vi "Stop Core.vi"(10 "final error code":i32, 11 "Error Reporter in":refnum<class "Error Reporter.lvclass">) -> (3 "Error Reporter out":refnum<class "Error Reporter.lvclass">)   [LabVIEW 2024, in "Error Reporting Actor.lvlib" / "Error Reporter.lvlib" / "Error Reporter.lvclass"]
doc: "<p>(<strong>Filename</strong>: <span class=\"dnl\">Actor Framework.lvlib:Actor.lvclass:Stop Core.vi</span>)</p>\n<p>Defines what the actor does before it stops. Use the <strong>final error code</strong> input to determine whether the actor shut down in response to an error.</p>\n<p>By default, this method passes the Stop message along to all <a href=\"nihelplauncher://docs/csh?context=lvcore_lvcomm_af_launch_nested_actor\">auto-stop nested actors</a>. A descendant class may override this method to define additional behavior, such as shutting down any processes the actor initiated in its override of the <a href=\"nihelplauncher://docs/csh?context=lvcore_lvcomm_af_actor_core\">Actor Core</a> method.</p>"
uses:
  Error Reporter.lvclass
  Error Reporter.lvclass/Error Reporter.ctl
  <vilib>/ActorFramework/Message Enqueuer/Message Enqueuer.lvclass/Message Enqueuer.ctl
  <vilib>/ActorFramework/Message Enqueuer/Enqueue.vi
  <vilib>/ActorFramework/Stop Msg/Stop Msg.lvclass
  C:/Program Files (x86)/National Instruments/LabVIEW 2024/vi.lib/ActorFramework/Message/Message.lvclass
  <vilib>/ActorFramework/Message Priority Queue/Priority Enqueue.vi
  <vilib>/ActorFramework/Actor/Actor.lvclass
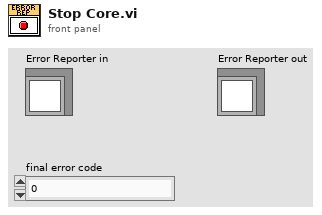
[diagram p1: front panel]
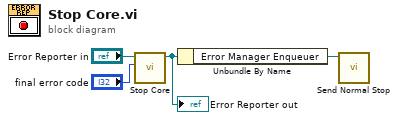
[diagram p0: block diagram]
diagram:
  n1 = call-parent "Stop Core.vi"("final error code"="final error code", "Actor in"="Error Reporter in") -> ("Actor out"=w2:refnum<class "Error Reporter.lvclass">)  [unwired: 9 in]
  "Error Reporter out" <- w2
  n2 = Unbundle By Name(w2) -> ("Error Manager Enqueuer"=w1:refnum<class "Message Enqueuer.lvclass">)
  n3 = call <vilib>:"Send Normal Stop.vi"("Message Enqueuer"=w1) -> ()  [unwired: 10 in, 1 out]
